vi "Finish.vi"   [LabVIEW 2013]
doc: "This VI is called just before exiting. It is expected to close I/O refnum, save collected data, etc."
uses:
  <vilib>/Rock Robotics/WPI/RobotDrive/WPI_RobotDriveGetSetRefNum.vi
  <vilib>/Rock Robotics/WPI/Joystick/WPI_JoystickGetSetRefNum.vi
types:
  T1 = typedef "WPI_JoystickDevRef.ctl" = cluster{"Device":T2}
  T2 = typedef "WPI_JoystickDeviceEnum.ctl" = enum16{"USB 1", "USB 2", "USB 3", "USB 4", "Kinect 1", "Kinect 2"}
  T3 = typedef "WPI_RobotDriveDevRef.ctl" = cluster{"DevStatus":errorcluster, "Motors[]":T4[], "Square Inputs":bool, "Max Output":dbl, "Isochronous":bool}
  T4 = typedef "WPI_MotorControlDeviceRef.ctl" = cluster{"DeviceStatus":errorcluster, "Type":enum16{"PWM", "CAN"}, "PWM":cluster{"Digital Module":T5, "PWM Channel":T6, "DeadBand":T7}, "CAN":cluster{"Device Number":u8, "Control Mode":T8, "Semaphore":T9, "Max Vout":dbl}, "Invert":bool, "TransformRef":T10, "InvTransformRef":T10}
  T5 = typedef "FPGA_TypedefDigitalModule.ctl" = enum16{"Digital Module 1", "Digital Module 2"}
  T6 = typedef "FPGA_DIOPWMChannel.ctl" = enum8{"PWM 1", "PWM 2", "PWM 3", "PWM 4", "PWM 5", "PWM 6", "PWM 7", "PWM 8", "PWM 9", "PWM 10", "Invalid"}
  T7 = typedef "WPI_PWMDeadband.ctl" = cluster{"Name":string, "maxPositivePwm":i32, "minPositivePwm":i32, "centerPwm":i32, "maxNegativePwm":i32, "minNegativePwm":i32, "angularRange":u16}
  T8 = typedef "WPI_CANJaguar_ControlMode.ctl" = enum8{"Percent VBus", "Current", "Speed", "Position", "Voltage"}
  T9 = typedef "Semaphore RefNum" = refnum<k1>
  T10 = typedef "WPI_PWMTransform_ConPane.ctl" = refnum<vi>
  T11 = typedef "WPI_RelayDevRef.ctl" = cluster{"DevStatus":errorcluster, "Relay Channel":T12, "Digital Module":T5, "Relay Direction":T13}
  T12 = typedef "FPGA_DIORelayChannel.ctl" = enum8{"Relay 1", "Relay 2", "Relay 3", "Relay 4", "Relay 5", "Relay 6", "Relay 7", "Relay 8", "Invalid"}
  T13 = typedef "WPI_RelayDirection.ctl" = enum16{"Both directions", "Forward only", "Reverse only"}
  T14 = typedef "WPI_AnalogChannelDevRef.ctl" = cluster{"DevStatus":errorcluster, "Analog Module":T15, "Analog Channel":T16}
  T15 = typedef "FPGA_TypedefAnalogModule.ctl" = enum16{"Analog Module 1", "Analog Module 2"}
  T16 = typedef "FPGA_AIChannel.ctl" = enum8{"AI 1", "AI 2", "AI 3", "AI 4", "AI 5", "AI 6", "AI 7", "AI 8", "Invalid"}
  T17 = typedef "WPI_SolenoidDevRef.ctl" = cluster{"DevStatus":errorcluster, "Solenoid Module":T18, "Forward Solenoid Channel":T19, "Reverse Solenoid Channel":T19}
  T18 = typedef "FPGA_TypedefSolenoidModule.ctl" = enum16{"Solenoid Module 1", "Solenoid Module 2"}
  T19 = typedef "WPI_SolenoidChannel.ctl" = enum8{"Solenoid 1", "Solenoid 2", "Solenoid 3", "Solenoid 4", "Solenoid 5", "Solenoid 6", "Solenoid 7", "Solenoid 8", "Invalid"}
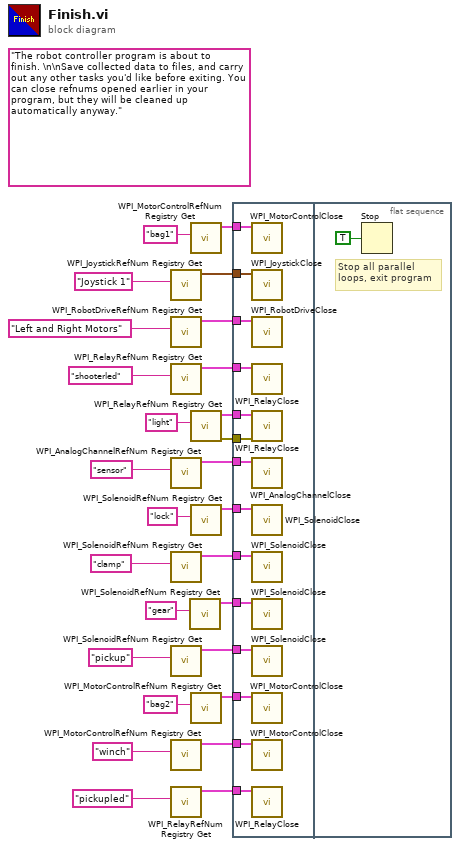
[diagram p0: block diagram]
diagram:
  (unwired) "The robot controller program is about to finish. \n\nSave collected data to files, and carry out any other tasks you'd like before exiting. You can close refnums opened earlier in your program, but they will be cleaned up automatically anyway."
  n1 = call <vilib>:"WPI_JoystickRefNum Registry Get.vi"("refnum name"="Joystick 1") -> ("JoystickDevRef"=w24:T1)  [unwired: 1 in, 9 out]
  n2 = call <vilib>:"WPI_RobotDriveRefNum Registry Get.vi"("refnum name"="Left and Right Motors") -> ("RobotDriveDevRef"=w25:T3)  [unwired: 1 in, 9 out]
  n3 = call <vilib>:"WPI_RelayRefNum Registry Get.vi"("refnum name"="shooterled") -> ("RelayDevRef"=w19:T11)  [unwired: 9 in, 1 out]
  n4 = call <vilib>:"WPI_AnalogChannelRefNum Registry Get.vi"("refnum name"="sensor") -> ("AIDeviceRef"=w5:T14)  [unwired: 9 in, 1 out]
  n5 = call <vilib>:"WPI_SolenoidRefNum Registry Get.vi"("refnum name"="clamp") -> ("SolenoidDevRef"=w10:T17)  [unwired: 9 in, 1 out]
  n6 = call <vilib>:"WPI_SolenoidRefNum Registry Get.vi"("refnum name"="pickup") -> ("SolenoidDevRef"=w11:T17)  [unwired: 9 in, 1 out]
  n7 = call <vilib>:"WPI_MotorControlRefNum Registry Get.vi"("refnum name"="winch") -> ("MotorControlDevRef"=w14:T4)  [unwired: 9 in, 1 out]
  n8 = call <vilib>:"WPI_RelayRefNum Registry Get.vi"("refnum name"="pickupled") -> ("RelayDevRef"=w18:T11)  [unwired: 9 in, 1 out]
  n9 = call <vilib>:"WPI_SolenoidRefNum Registry Get.vi"("refnum name"="gear") -> ("SolenoidDevRef"=w13:T17)  [unwired: 9 in, 1 out]
  n10 = call <vilib>:"WPI_MotorControlRefNum Registry Get.vi"("refnum name"="bag1") -> ("MotorControlDevRef"=w23:T4)  [unwired: 9 in, 1 out]
  n11 = call <vilib>:"WPI_RelayRefNum Registry Get.vi"("refnum name"="light") -> ("error out"=w2:errorcluster, "RelayDevRef"=w3:T11)  [unwired: 9 in]
  n12 = call <vilib>:"WPI_SolenoidRefNum Registry Get.vi"("refnum name"="lock") -> ("SolenoidDevRef"=w12:T17)  [unwired: 9 in, 1 out]
  n13 = call <vilib>:"WPI_MotorControlRefNum Registry Get.vi"("refnum name"="bag2") -> ("MotorControlDevRef"=w22:T4)  [unwired: 9 in, 1 out]
  n14 = flat-sequence {
    tunnel: w25 -> [w41]
    tunnel: w24 -> [w40]
    tunnel: w23 -> [w39]
    tunnel: w22 -> [w38]
    tunnel: w19 -> [w37]
    tunnel: w18 -> [w36]
    tunnel: w14 -> [w35]
    tunnel: w13 -> [w34]
    tunnel: w12 -> [w33]
    tunnel: w11 -> [w32]
    tunnel: w10 -> [w31]
    tunnel: w5 -> [w30]
    tunnel: w3 -> [w29]
    tunnel: w2 -> [w28]
    frame #0 {
      n15 = call <vilib>:"WPI_MotorControlClose.vi"("MotorControlDevRef"=w39) -> ()  [unwired: 10 in, 1 out]
      n16 = call <vilib>:"WPI_JoystickClose.vi"("JoystickDevRef"=w40) -> ()  [unwired: 11 out]
      n17 = call <vilib>:"WPI_RobotDriveClose.vi"("RobotDriveDevRef"=w41) -> ()  [unwired: 1 in, 10 out]
      n18 = call <vilib>:"WPI_RelayClose.vi"("RelayDevRef"=w37) -> ()  [unwired: 10 in, 1 out]
      n19 = call <vilib>:"WPI_RelayClose.vi"("error in (no error)"=w28, "RelayDevRef"=w29) -> ()  [unwired: 9 in, 1 out]
      n20 = call <vilib>:"WPI_AnalogChannelClose.vi"("AIDeviceRef"=w30) -> ()  [unwired: 10 in, 1 out]
      n21 = call <vilib>:"WPI_SolenoidClose.vi"("SolenoidDevRef"=w33) -> ()  [unwired: 10 in, 1 out]
      n22 = call <vilib>:"WPI_SolenoidClose.vi"("SolenoidDevRef"=w31) -> ()  [unwired: 10 in, 1 out]
      n23 = call <vilib>:"WPI_SolenoidClose.vi"("SolenoidDevRef"=w34) -> ()  [unwired: 10 in, 1 out]
      n24 = call <vilib>:"WPI_SolenoidClose.vi"("SolenoidDevRef"=w32) -> ()  [unwired: 10 in, 1 out]
      n25 = call <vilib>:"WPI_MotorControlClose.vi"("MotorControlDevRef"=w38) -> ()  [unwired: 10 in, 1 out]
      n26 = call <vilib>:"WPI_MotorControlClose.vi"("MotorControlDevRef"=w35) -> ()  [unwired: 10 in, 1 out]
      n27 = call <vilib>:"WPI_RelayClose.vi"("RelayDevRef"=w36) -> ()  [unwired: 10 in, 1 out]
    }
    frame #1 {
      # "Stop all parallel\nloops, exit program"
      n28 = Stop(stop? (T)=TRUE ("Quit")) -> ()
    }
  }
